vi "DEC to BCD.vi"(11 "DEC":i32) -> (3 "BCD":u8)   [LabVIEW 2011, in "LMH-Toolbox.lvlib" / "LMH-Common.lvlib"]
doc: "Convert a decimal number to a binary coded decimal."
uses:
  LMH-Common.lvlib
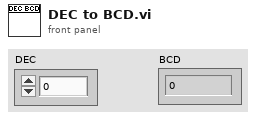
[diagram p1: front panel]
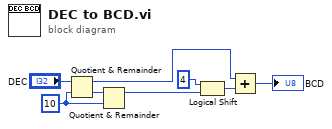
[diagram p0: block diagram]
diagram:
  w6 = 10 ("y")
  n1 = Quotient & Remainder(x="DEC", y=w6) -> (x-y*floor(x/y)=w2:i32, floor(x/y)=w7:i32)
  n2 = Quotient & Remainder(x=w7, y=w6) -> (x-y*floor(x/y)=w5:i32)  [unwired: 1 out]
  n3 = Logical Shift(y=i8 4, x=w5) -> (x << y=w3:i32)
  n4 = Add(x=w2, y=w3) -> (x+y=→"BCD":i32)
